vi "Update Property.vi"(8 "error in (no error)":errorcluster, 9 "Value":variant, 10 "Name":string, 11 "StringPanel in":refnum<class "StringPanel.lvclass">) -> (0 "error out":errorcluster, 3 "StringPanel out":refnum<class "StringPanel.lvclass">)   [LabVIEW 2020, in "Conditum-Tools.lvlib" / "StringPanel.lvclass"]
uses:
  StringPanel.lvclass
  StringPanel.lvclass/StringPanel.ctl
  Conditum-Clone/Columns/String/String.lvclass
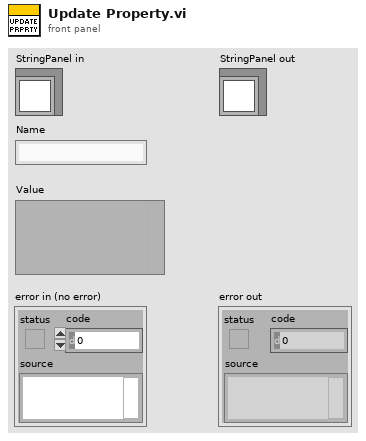
[diagram p1: front panel]
types:
  T1 = typedef "Conditu2.lvlib/Columns.lvlib/String.lvclass/Definition.ctl" = cluster{"Default":string, "Length":i32}
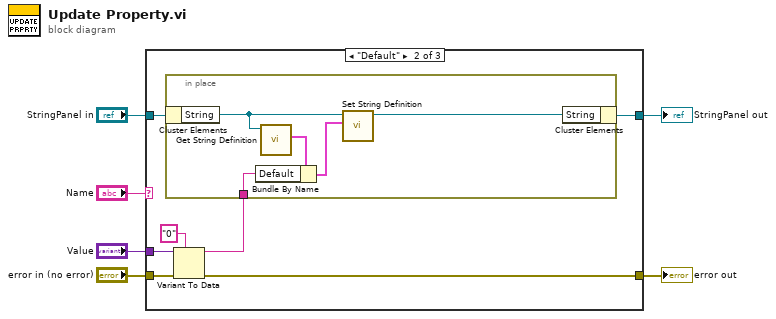
[diagram p0: block diagram]
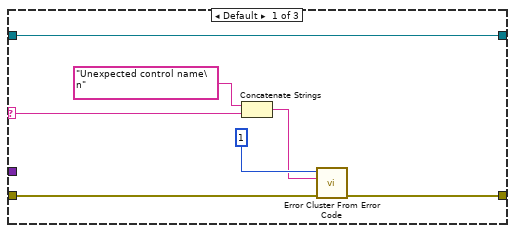
[diagram p2: hidden frame]
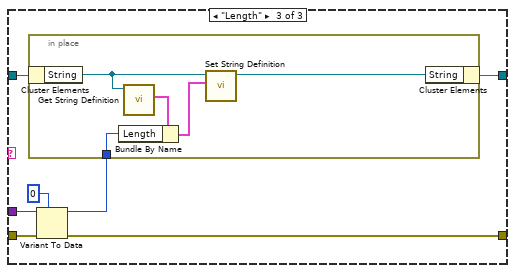
[diagram p3: hidden frame]
diagram:
  n1 = case shown="\"Default\"" "Name" {
    selector: "Name" -> [w9 _ _]
    tunnel: "Value" -> [_ w20 w32]
    tunnel: "StringPanel in" -> [w7 w16 w28]
    tunnel: "error in (no error)" -> [w13 w18 w30]
    tunnel: [w12 w17 w29] -> w4
    tunnel: [w7 w14 w26] -> w5
    frame Default {
      n2 = Concatenate Strings("Unexpected control name\n" ("format string"), w9) -> (w8:string)
      n3 = call <vilib>:"Error Cluster From Error Code.vi"("error in (no error)"=w13, "error message (\"\")"=w8, "error code (0)"=1) -> ("error out"=w12:errorcluster)  [unwired: 6 in]
    }
    frame "Default" {
      n4 = Variant To Data(error in=w18, type="0", Variant=w20) -> (data=w15:string, error out=w17:errorcluster)
      n5 = in-place {
        in-place-border: w15 -> [w24]
        n6 = in-place-cluster #1(w16) -> ("String"=w23:refnum<class "String.lvclass">)
        n7 = call "Get String Definition.vi"("String in"=w23) -> ("Definition"=w25:T1)  [unwired: 10 in]
        n8 = Bundle By Name(cluster=w25, "Default"=w24) -> (w22:T1)
        n9 = call "Set String Definition.vi"("String Definition"=w22, "String in"=w23) -> ("String out"=w21:refnum<class "String.lvclass">)  [unwired: 9 in]
        n10 = in-place-cluster #1("String"=w21) -> (w14:refnum<class "StringPanel.lvclass">)
      }
    }
    frame "Length" {
      n11 = Variant To Data(error in=w30, type=0, Variant=w32) -> (data=w27:i32, error out=w29:errorcluster)
      n12 = in-place {
        in-place-border: w27 -> [w36]
        n13 = in-place-cluster #2(w28) -> ("String"=w35:refnum<class "String.lvclass">)
        n14 = call "Get String Definition.vi"("String in"=w35) -> ("Definition"=w37:T1)  [unwired: 10 in]
        n15 = Bundle By Name(cluster=w37, "Length"=w36) -> (w34:T1)
        n16 = call "Set String Definition.vi"("String Definition"=w34, "String in"=w35) -> ("String out"=w33:refnum<class "String.lvclass">)  [unwired: 9 in]
        n17 = in-place-cluster #2("String"=w33) -> (w26:refnum<class "StringPanel.lvclass">)
      }
    }
  }
  "error out" <- w4
  "StringPanel out" <- w5
